vi "MaxiGauge_Main_Panel.vi"() -> ()   [LabVIEW 2019]
panel:
  out "GAUGE  Status: (Channel 1, 2, 3, 4, 5, 6, )":string
  in  "Channel 6":enum16{"NO CHANGE", "OFF", "ON"}(ring)
  in  "Channel 5":enum16{"NO CHANGE", "OFF", "ON"}(ring)
  in  "Channel 4":enum16{"NO CHANGE", "OFF", "ON"}(ring)
  in  "Channel 3":enum16{"NO CHANGE", "OFF", "ON"}(ring)
  in  "Channel 2":enum16{"NO CHANGE", "OFF", "ON"}(ring)
  in  "Channel 1":enum16{"NO CHANGE", "OFF", "ON"}(ring)
  in  "Gauge On/Off/Status":bool
  out "Sensor Type: (Channel 1, 2, 3, 4, 5, 6, )":string
  in  "Get Pressure sensor type":bool
  in  "Maxi_visa":refnum<visa-resource-name>
  in  "Measurement Rate (ms)":i32
  out "Channel 6":string
  out "Channel 5":string
  out "Channel 4":string
  out "Channel 3":string
  out "Channel 2":string
  out "Channel 1":string
  # "Gauge On/Off/Status"
  # "Pressure Value\n(Torr)"
  # "Gauge status:\n1 = OFF\n2 = ON"
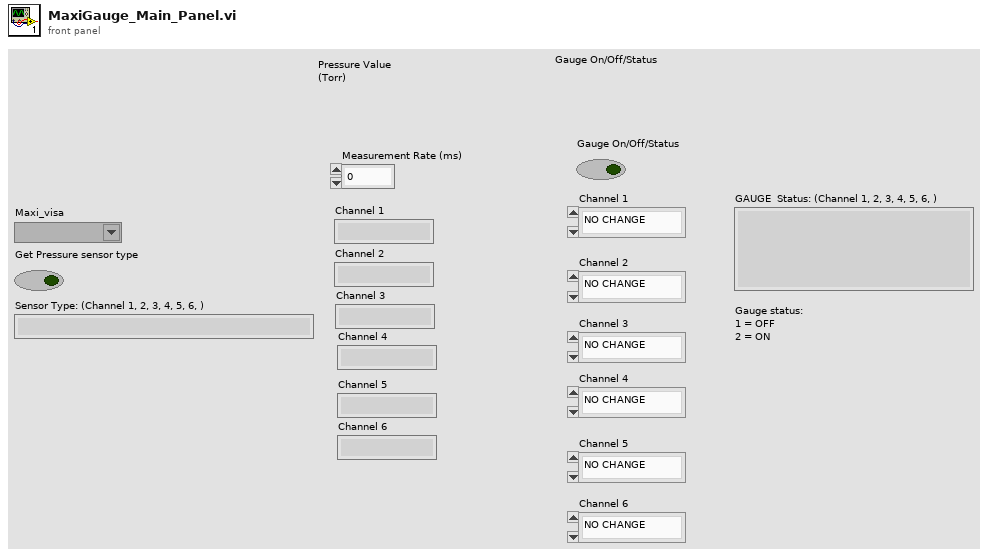
[diagram p1: front panel]
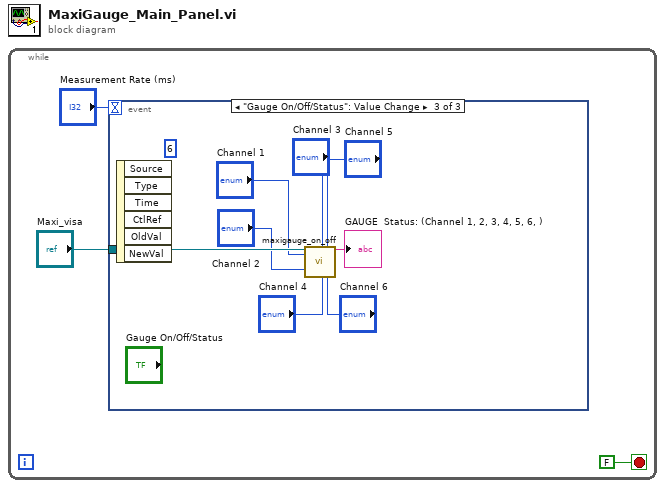
[diagram p0: block diagram]
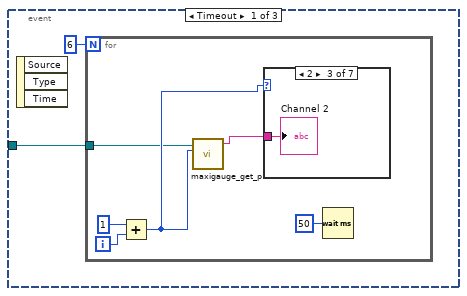
[diagram p2: hidden frame]
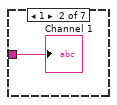
[diagram p4: hidden frame]
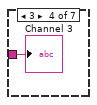
[diagram p5: hidden frame]
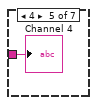
[diagram p6: hidden frame]
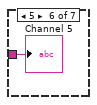
[diagram p7: hidden frame]
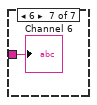
[diagram p8: hidden frame]
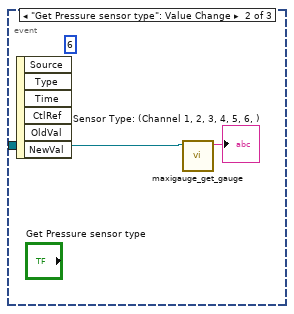
[diagram p9: hidden frame]
diagram:
  n1 = while {
    stop <- FALSE stop-if-true
    n2 = event shown="[2] \"Gauge On/Off/Status\": Value Change" {
      selector: _ -> [_ _ _]
      dyn-events: _ -> [_ _ _]
      timeout: "Measurement Rate (ms)" -> [_ _ _]
      tunnel: "Maxi_visa" -> [w4 w19 w27]
      event Timeout {
        n3 = event-data() -> ()  [unwired: 1 in, 3 out]
        n4 = for {
          N: 6 -> [_]
          tunnel: w4 -> [w6]
          i -> [w11]
          n5 = Add(x=1, y=w11) -> (x+y=w8:i32)
          n6 = call "maxigauge_get_p.vi"(9:w8, "maxi_visa"=w6) -> ("Pressure (Torr)"=w7:string)  [unwired: 7 in, 1 out]
          n7 = case shown="2" w8 {
            tunnel: w7 -> [_ w12 w13 w14 w15 w16 w17]
            frame 0, Default {
            }
            frame 1 {
              "Channel 1" <- w12
            }
            frame 2 {
              "Channel 2" <- w13
            }
            frame 3 {
              "Channel 3" <- w14
            }
            frame 4 {
              "Channel 4" <- w15
            }
            frame 5 {
              "Channel 5" <- w16
            }
            frame 6 {
              "Channel 6" <- w17
            }
          }
          n8 = Wait (ms)(milliseconds to wait=u32 50) -> ()  [unwired: 1 out]
        }
      }
      event "Get Pressure sensor type": Value Change {
        (unwired) 6
        n9 = event-data() -> ()  [unwired: 1 in, 6 out]
        n10 = call "maxigauge_get_gauge.vi"("maxi_visa"=w19) -> ("Gauge Type"=→"Sensor Type: (Channel 1, 2, 3, 4, 5, 6, )":string)  [unwired: 8 in, 1 out]
      }
      event "Gauge On/Off/Status": Value Change {
        (unwired) 6
        n11 = event-data() -> ()  [unwired: 1 in, 6 out]
        n12 = call "maxigauge_on_off.vi"("maxi_visa"=w27, "Channel 1"="Channel 1", "Channel 2"="Channel 2", "Channel 3"="Channel 3", "Channel 4"="Channel 4", "Channel 5"="Channel 5", "Channel 6"="Channel 6") -> ("GAUGE  Status"=→"GAUGE  Status: (Channel 1, 2, 3, 4, 5, 6, )":string)  [unwired: 11 in, 1 out]
      }
    }
  }
